vi "databasesync.vi"   [LabVIEW 2016, in "数据查询.lvlib"]
uses:
  <vilib>/Utility/sysdir.llb/System Directory Type.ctl
types:
  T1 = typedef "数据库类型.ctl" = enum16{"Access", "SQLite"}
  T2 = typedef "System Directory Type.ctl" = i32
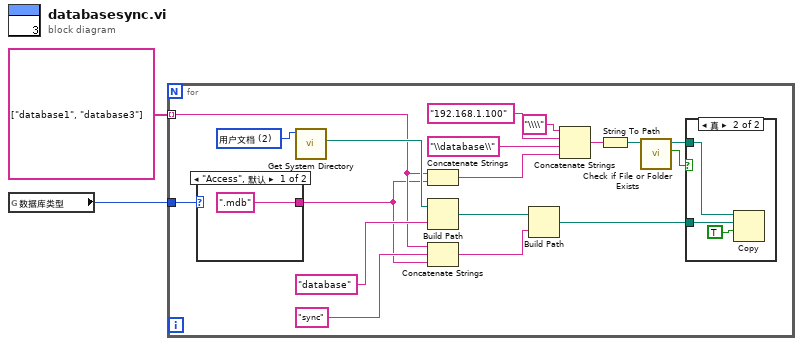
[diagram p0: block diagram]
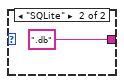
[diagram p3: hidden frame]
diagram:
  n1 = global read "外部调用接口全局变量.vi" "数据库类型"() -> (w1:T1)
  n2 = for {
    tunnel: string[] ["database1", "database3"] -> [w10] mode=indexing
    tunnel: w1 -> [w20]
    w14 = T2 2 items=["用户目录"=0, "用户桌面"=1, "用户文档"=2, "用户应用程序数据"=3, "用户设置"=4, "用户临时目录"=5, "公共文档"=6, "公共应用程序数据"=7, "公共设置"=8, "公共缓存"=13, "系统核心库"=9, "系统安装库"=10, "应用程序文件"=11, "启动盘根目录"=12] ("system directory type")
    n3 = case shown="\"Access\", 默认" w20 {
      tunnel: [".mdb" ".db"] -> w8
      frame "Access", Default {
      }
      frame "SQLite" {
      }
    }
    n4 = call <vilib>:"Get System Directory.vi"("system directory type"=w14) -> ("system directory"=w15:path)  [unwired: 10 in]
    n5 = Concatenate Strings(w10, w8) -> (w11:string)
    n6 = Build Path(base path=w15, name or relative path="database" ("名称或相对路径")) -> (appended path=w12:path)
    n7 = Concatenate Strings(w10, "sync" ("字符串"), w8) -> (w7:string)
    n8 = Build Path(base path=w12, name or relative path=w7) -> (appended path=w6:path)
    n9 = Concatenate Strings("\\\\" ("字符串"), "192.168.1.100" ("名称"), "\\database\\" ("字符串"), w11) -> (w18:string)
    n10 = String To Path(string=w18) -> (path=w5:path)
    n11 = call <vilib>:"Check if File or Folder Exists.vi"("path"=w5) -> ("file or folder exists?"=w4:bool, "dup path"=w3:path)  [unwired: 8 in, 1 out]
    n12 = case shown="真" w4 {
      tunnel: w6 -> [_ w23]
      tunnel: w3 -> [_ w21]
      frame False {
      }
      frame True {
        n13 = Copy(9:TRUE ("覆盖(F)"), 10:w23, 11:w21) -> ()  [unwired: 2 in, 3 out]
      }
    }
  }
